vi "Float64Array Create.vi"(8 "error in (no error)":errorcluster, 11 "DBL array in":dbl[](array[numeric])) -> (0 "error out":errorcluster, 3 "Float64Array DVR out":refnum<data-value>)   [LabVIEW 2012, in "MDSplus.lvlib"]
uses:
  <vilib>/MDSplus/Library/MDSplus.lvlib
  <vilib>/MDSplus/Classes/Data_Class/Array_Class/Float64Array_Class/Float64Array.lvclass
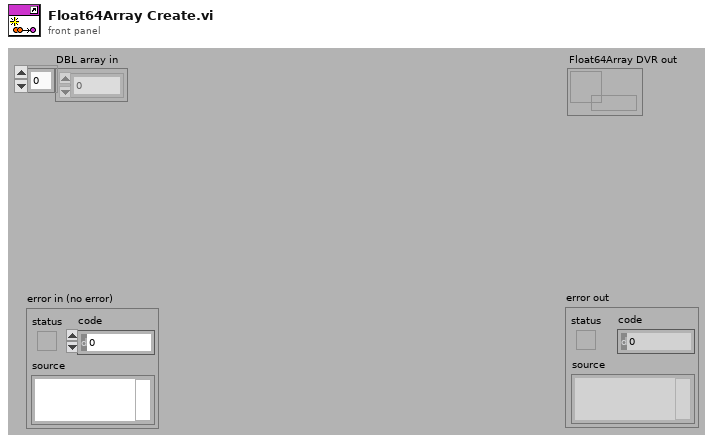
[diagram p1: front panel]
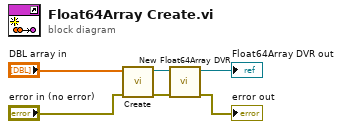
[diagram p0: block diagram]
diagram:
  n1 = call <vilib>:"Create.vi"("error in (no error)"="error in (no error)", "DBL array in"="DBL array in") -> ("error out"=w3:errorcluster, "Float64Array out"=w4:refnum<class "Float64Array.lvclass">)  [unwired: 8 in]
  n2 = call <vilib>:"New Float64Array DVR.vi"("error in (no error)"=w3, "Float64Array in"=w4) -> ("error out"=→"error out":errorcluster, "Float64Array DVR out"=→"Float64Array DVR out":refnum<data-value>)  [unwired: 8 in]
